vi "Get All Property Names.vi"(8 "error in":errorcluster, 11 "Item Ref in":refnum<data-value>) -> (0 "error out":errorcluster, 3 "Property Names":string[](array[string]))   [LabVIEW 2024, in "Config File Parser.lvlib" / "Property.lvclass"]
uses:
  Property.lvclass
  Item/Item.lvclass
  Property.lvclass/Property.ctl
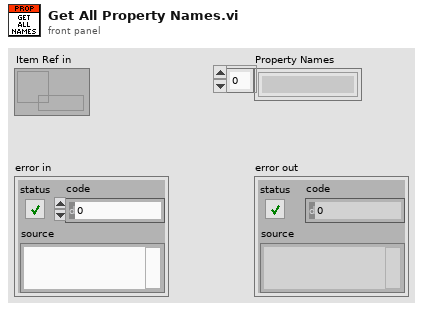
[diagram p1: front panel]
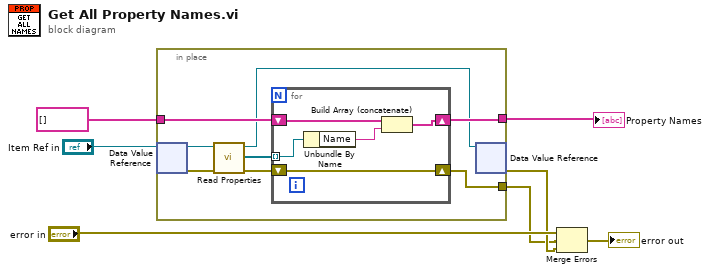
[diagram p0: block diagram]
diagram:
  n1 = in-place "In Place Element Structure" {
    in-place-border: string[] [] -> [w10]
    in-place-border: [w13] -> w4
    in-place-border: [w9] -> w1
    n2 = in-place-dvr #1("Item Ref in") -> (w12:refnum<class "Item.lvclass">, w15:errorcluster)
    n3 = call-dynamic "Read Properties.vi"("error in (no error)"=w15, "Item in"=w12) -> ("error out"=w14:errorcluster, "Properties"=w11:refnum<class "Property.lvclass">[], "Item out"=w8:refnum<class "Item.lvclass">)  [unwired: 7 in]
    n4 = for {
      tunnel: w11 -> [w19] mode=indexing
      shift-right: [w20] -> w13
      shift-left: w14 -> [w20]
      shift-right: [w17] -> w9
      shift-left: w10 -> [w18]
      n5 = Unbundle By Name(w19) -> ("Name"=w16:string)
      n6 = Build Array (concatenate)(w18, w16) -> (w17:string[])
    }
    n7 = in-place-dvr #1(w8) -> (w6:errorcluster)  [unwired: 1 out]
  }
  "Property Names" <- w1
  n8 = Merge Errors("error in", w4, w6) -> (→"error out":errorcluster)
